vi "fg.vi"() -> (2 "波形数据":dbl[](array[numeric]) format="%.2f", 3 "波形数据 2":dbl[](array[numeric]) format="%.2f", 4 "Numeric":dbl format="%.2f")   [LabVIEW 2010]
uses:
  <vilib>/Analysis/NI_AALBase.lvlib
panel:
  in  "宽 度":dbl format="%.2f"
  in  "延 时":dbl format="%.2f"
  in  "宽 度":dbl format="%.2f"
  in  "延 时":dbl format="%.2f"
  in  "方波周期 2":dbl=50.0 format="%.2f"
  in  "重置相位":bool=TRUE
  in  "方波周期":dbl=50.0 format="%.2f"
  in  "重置相位":bool=TRUE
  in  "ºÏ³É   ·ÖÀë ·":bool=TRUE
  in  "频   率":dbl(slide)=50.0 scale=0.0..5000.0
  in  "信号类型":u16(ring) items=["正弦波", "方波", "三角波", "均匀白噪声", "脉冲函数"]
  in  "幅 值":dbl=5.0 format="%.2f"
  in  "偏 置":dbl format="%.2f"
  in  "相 位":dbl format="%.2f"
  in  "取样率":dbl=4096.0 format="%.2f"
  in  "频  率":dbl(slide)=100.0 scale=0.0..5000.0
  in  "波    形":u16(ring) items=["正弦波", "方波", "三角波", "均匀白噪声", "脉冲函数", "冲激函数"]
  in  "幅 值":dbl=5.0 format="%.2f"
  in  "偏 置":dbl format="%.2f"
  in  "相 位":dbl format="%.2f"
  # "多通道信号发生器"
  # "一\n信\n道"
  # "二 \n信\n道"
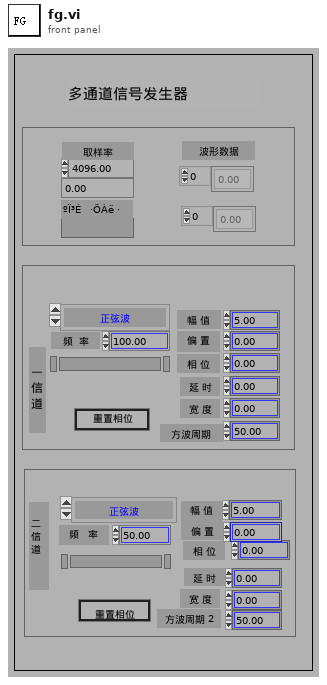
[diagram p1: front panel]
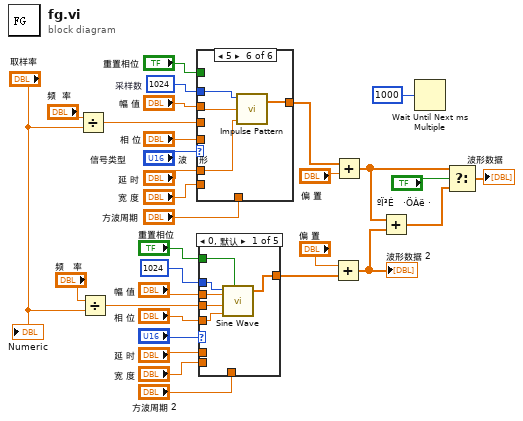
[diagram p0: block diagram]
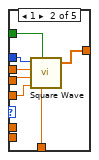
[diagram p2: hidden frame]
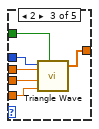
[diagram p3: hidden frame]
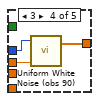
[diagram p4: hidden frame]
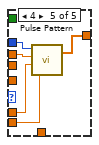
[diagram p5: hidden frame]
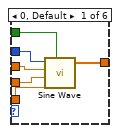
[diagram p6: hidden frame]
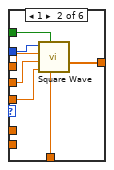
[diagram p7: hidden frame]
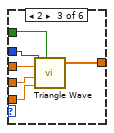
[diagram p8: hidden frame]
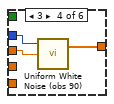
[diagram p9: hidden frame]
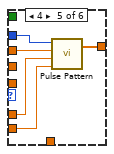
[diagram p10: hidden frame]
diagram:
  w24 = 1024  # 采样数
  n1 = Divide(x="频  率", y="取样率") -> (x/y=w28:dbl)
  n2 = Divide(x="频   率", y="取样率") -> (x/y=w13:dbl)
  n3 = case shown="5" "波    形" {
    tunnel: "幅 值" -> [w35 w38 w49 w51 w56 w60]
    tunnel: w28 -> [w37 w39 w48 _ _ _]
    tunnel: [w36 w44 w50 w52 w58 w62] -> w6
    tunnel: "相 位" -> [w34 w43 w47 _ _ _]
    tunnel: w24 -> [w33 w42 w46 w53 w57 w61]
    tunnel: "方波周期" -> [_ w41 _ _ _ _]
    tunnel: "重置相位" -> [w32 w40 w45 _ _ _]
    tunnel: "延 时" -> [_ _ _ _ w55 w59]
    tunnel: "宽 度" -> [_ _ _ _ w54 _]
    frame 0, Default {
      n4 = call <vilib>:"Sine Wave.vi"("samples"=w33, "amplitude"=w35, "frequency"=w37, "phase in"=w34, "reset phase"=w32) -> ("sine wave"=w36:dbl[])  [unwired: 2 out]
    }
    frame 1 {
      n5 = call <vilib>:"Square Wave.vi"("samples"=w42, "reset phase"=w40, "amplitude"=w38, "frequency"=w39, "duty cycle (%)"=w41, "phase in"=w43) -> ("square wave"=w44:dbl[])  [unwired: 2 out]
    }
    frame 2 {
      n6 = call <vilib>:"Triangle Wave.vi"("samples"=w46, "amplitude"=w49, "frequency"=w48, "phase in"=w47, "reset phase"=w45) -> ("triangle wave"=w50:dbl[])  [unwired: 2 out]
    }
    frame 3 {
      n7 = call <vilib>:"Uniform White Noise (obs 90).vi"("amplitude"=w51, "samples"=w53) -> ("uniform white noise"=w52:dbl[])  [unwired: 1 in, 1 out]
    }
    frame 4 {
      n8 = call <vilib>:"Pulse Pattern.vi"("width"=w54, "delay"=w55, "amplitude"=w56, "samples"=w57) -> ("Pulse Pattern"=w58:dbl[])  [unwired: 1 out]
    }
    frame 5 {
      n9 = call <vilib>:"Impulse Pattern.vi"("delay"=w59, "amplitude"=w60, "samples"=w61) -> ("Impulse Pattern"=w62:dbl[])  [unwired: 1 out]
    }
  }
  n10 = case shown="0, 默认" "信号类型" {
    tunnel: "幅 值" -> [w66 w74 w80 w82 w87]
    tunnel: w13 -> [w68 w73 w79 _ _]
    tunnel: [w67 w75 w81 w83 w89] -> w16
    tunnel: "相 位" -> [w65 w72 w78 _ _]
    tunnel: 1024 -> [w64 w71 w77 w84 w88]
    tunnel: "重置相位" -> [w63 w69 w76 _ _]
    tunnel: "方波周期 2" -> [_ w70 _ _ _]
    tunnel: "延 时" -> [_ _ _ _ w86]
    tunnel: "宽 度" -> [_ _ _ _ w85]
    frame 0, Default {
      n11 = call <vilib>:"Sine Wave.vi"("samples"=w64, "amplitude"=w66, "frequency"=w68, "phase in"=w65, "reset phase"=w63) -> ("sine wave"=w67:dbl[])  [unwired: 2 out]
    }
    frame 1 {
      n12 = call <vilib>:"Square Wave.vi"("samples"=w71, "reset phase"=w69, "amplitude"=w74, "frequency"=w73, "duty cycle (%)"=w70, "phase in"=w72) -> ("square wave"=w75:dbl[])  [unwired: 2 out]
    }
    frame 2 {
      n13 = call <vilib>:"Triangle Wave.vi"("samples"=w77, "amplitude"=w80, "frequency"=w79, "phase in"=w78, "reset phase"=w76) -> ("triangle wave"=w81:dbl[])  [unwired: 2 out]
    }
    frame 3 {
      n14 = call <vilib>:"Uniform White Noise (obs 90).vi"("amplitude"=w82, "samples"=w84) -> ("uniform white noise"=w83:dbl[])  [unwired: 1 in, 1 out]
    }
    frame 4 {
      n15 = call <vilib>:"Pulse Pattern.vi"("width"=w85, "delay"=w86, "amplitude"=w87, "samples"=w88) -> ("Pulse Pattern"=w89:dbl[])  [unwired: 1 out]
    }
  }
  n16 = Add(x="偏 置", y=w16) -> (x+y=w18:dbl[])
  "波形数据 2" <- w18
  n17 = Add(x=w6, y="偏 置") -> (x+y=w21:dbl[])
  n18 = Add(x=w21, y=w18) -> (x+y=w20:dbl[])
  n19 = Wait Until Next ms Multiple(millisecond multiple=u32 1000) -> ()  [unwired: 1 out]
  n20 = Select(t=w21, s="ºÏ³É   ·ÖÀë ·", f=w20) -> (s? t:f=→"波形数据":dbl[])
  "Numeric" <- "取样率"
